vi "TcA01-010_ExternalOwner.vi"(1 "occurrence":refnum<k4>, 5 "error in (no error)":errorcluster) -> (19 "error out":errorcluster)   [LabVIEW 2020]
uses:
  TestClasses/G#SubClass1_class/G#SubClass1.lvclass
  <vilib>/addons/_AddQ/G#Object/G#Object.lvclass
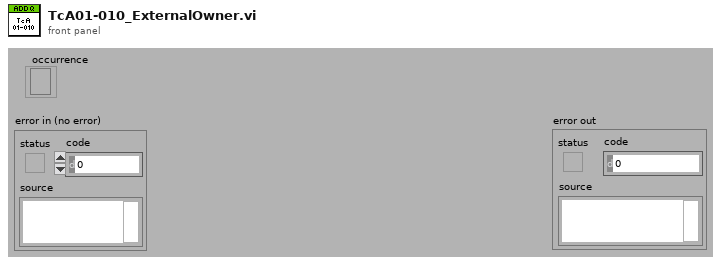
[diagram p1: front panel]
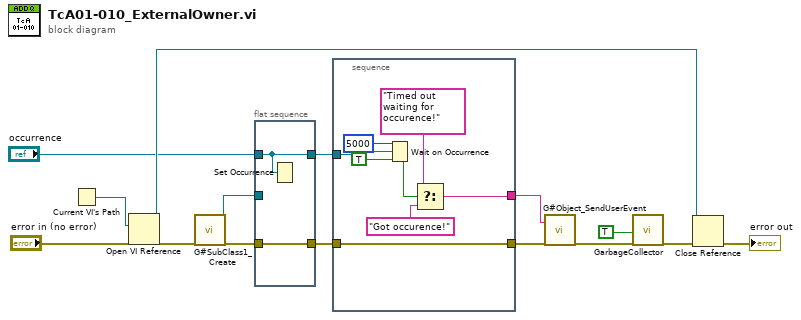
[diagram p0: block diagram]
diagram:
  n1 = Current VI's Path() -> (path=w12:path)
  n2 = Open VI Reference(vi path=w12, error in (no error)="error in (no error)") -> (vi reference=w9:refnum<vi>, error out=w13:errorcluster)  [unwired: 4 in]
  n3 = call "G#SubClass1_Create.vi"("error in (no error)"=w13) -> ("reference out"=w1:refnum<class "G#SubClass1.lvclass">, "error out"=w3:errorcluster)  [unwired: 16 in, 1 out]
  n4 = flat-sequence {
    tunnel: [w16] -> w5
    tunnel: "occurrence" -> [w16]
    tunnel: w3 -> [w17]
    tunnel: [w17] -> w2
    tunnel: w1 -> [_]
    frame #0 {
      n5 = Set Occurrence(w16) -> ()
    }
  }
  n6 = stacked-sequence {
    tunnel: w2 -> [w22]
    tunnel: w5 -> [w23]
    tunnel: [w22] -> w8
    tunnel: [w18] -> w6
    frame #0 {
      n7 = Wait on Occurrence(1:TRUE ("ignore previous (T)"), 2:w23, 3:5000 ("ms timeout (-1)")) -> (0:w21:bool)
      n8 = Select(t="Timed out waiting for occurence!", s=w21, f="Got occurence!") -> (s? t:f=w18:string)
    }
  }
  n9 = call <vilib>:"G#Object_SendUserEvent.vi"("text"=w6, "error in (no error)"=w8) -> ("error out"=w7:errorcluster)  [unwired: 16 in, 1 out]
  n10 = call <vilib>:"GarbageCollector.vi"("only from same owner as caller? (T)"=TRUE ("only from same owner as caller?"), "error in (no error)"=w7) -> ("error out"=w11:errorcluster)  [unwired: 15 in, 2 out]
  n11 = Close Reference(reference=w9, error in (no error)=w11) -> (error out=→"error out":errorcluster)
